vi "Initialize Attributes.vi"(8 "error in (no error)":errorcluster, 10 "Attribute Data":variant, 11 "BNT_DSCXYGraph in":refnum<class "BNT_DSCXYGraph.lvclass">) -> (0 "error out":errorcluster, 2 "Found?":bool, 3 "BNT_DSCXYGraph out":refnum<class "BNT_DSCXYGraph.lvclass">)   [LabVIEW 2015, in "BNT_DSCXYGraph.lvlib" / "BNT_DSCXYGraph.lvclass"]
doc: "Initialize object attribute.\n\nUnique resources should be allocated elsewhere!"
uses:
  BNT_DSCXYGraph.lvclass
  BNT_DSCXYGraph.lvclass/BNT_DSCXYGraph.ctl
  CSPP_Core/Actors/CS++GUIActor/CS++GUIActor.lvclass
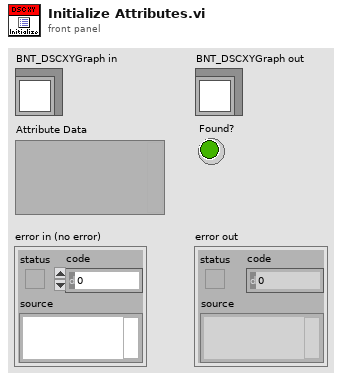
[diagram p1: front panel]
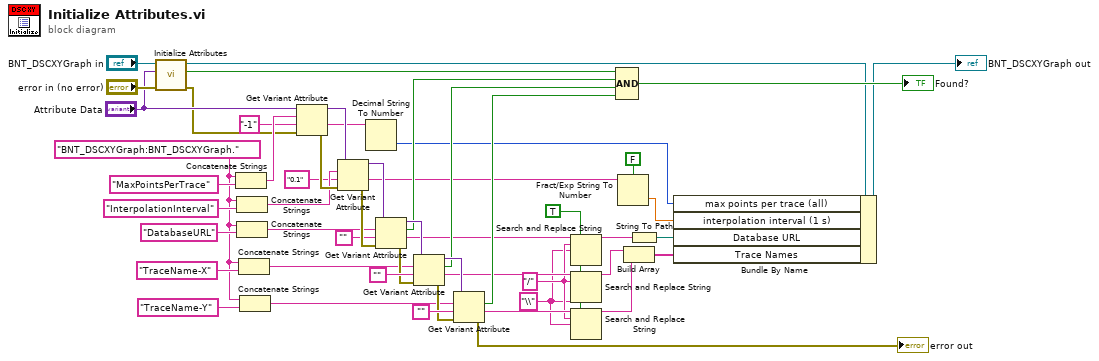
[diagram p0: block diagram]
diagram:
  w3 = TRUE ("replace all? (F)")
  w1 = "\\" ("replace string (\"\")")
  w2 = "/" ("search string")
  w38 = "BNT_DSCXYGraph:BNT_DSCXYGraph."
  n1 = call-parent "Initialize Attributes.vi"("error in (no error)"="error in (no error)", "Attribute Data"="Attribute Data", "CS++GUIActor in"="BNT_DSCXYGraph in") -> ("error out"=w44:errorcluster, "Found?"=w45:bool, "CS++GUIActor out"=w11:refnum<class "BNT_DSCXYGraph.lvclass">)  [unwired: 6 in]
  n2 = Concatenate Strings(w38, "MaxPointsPerTrace" ("string")) -> (w50:string)
  n3 = Concatenate Strings(w38, "InterpolationInterval" ("string")) -> (w47:string)
  n4 = Concatenate Strings(w38, "DatabaseURL" ("string")) -> (w33:string)
  n5 = Concatenate Strings(w38, "TraceName-X" ("string")) -> (w28:string)
  n6 = Concatenate Strings(w38, "TraceName-Y" ("string")) -> (w24:string)
  n7 = Get Variant Attribute(Variant="Attribute Data", name=w50, default value (empty Variant)="-1" ("string"), error in=w44) -> (duplicate Variant=w49:variant, value=w16:string, error out=w48:errorcluster)  [unwired: 1 out]
  n8 = Get Variant Attribute(Variant=w49, name=w47, default value (empty Variant)="0.1" ("string"), error in=w48) -> (duplicate Variant=w35:variant, value=w14:string, error out=w34:errorcluster)  [unwired: 1 out]
  n9 = Decimal String To Number(string=w16) -> (number=w15:i32)  [unwired: 2 in, 1 out]
  n10 = Get Variant Attribute(Variant=w35, name=w33, default value (empty Variant)="", error in=w34) -> (duplicate Variant=w30:variant, found=w23:bool, value=w4:string, error out=w29:errorcluster)
  n11 = Get Variant Attribute(Variant=w30, name=w28, default value (empty Variant)="", error in=w29) -> (duplicate Variant=w25:variant, found=w22:bool, value=w9:string, error out=w26:errorcluster)
  n12 = Get Variant Attribute(Variant=w25, name=w24, default value (empty Variant)="", error in=w26) -> (found=w21:bool, value=w7:string, error out=→"error out":errorcluster)  [unwired: 1 out]
  n13 = Search and Replace String(replace all?=w3, input string=w4, search string=w2, replace string=w1) -> (result string=w5:string)  [unwired: 4 in, 3 out]
  n14 = Search and Replace String(replace all?=w3, input string=w9, search string=w2, replace string=w1) -> (result string=w8:string)  [unwired: 4 in, 3 out]
  n15 = Search and Replace String(replace all?=w3, input string=w7, search string=w2, replace string=w1) -> (result string=w6:string)  [unwired: 4 in, 3 out]
  n16 = Compound Arithmetic op=AND(w45, w23, w22, w21) -> (→"Found?":bool)
  n17 = Fract/Exp String To Number(use system decimal point (T)=FALSE, string=w14) -> (number=w13:dbl)  [unwired: 2 in, 1 out]
  n18 = Build Array(w8, w6) -> (w17:string[])
  n19 = String To Path(string=w5) -> (path=w18:path)
  n20 = Bundle By Name(cluster=w11, "max points per trace (all)"=w15, "interpolation interval (1 s)"=w13, "Database URL"=w18, "Trace Names"=w17) -> (→"BNT_DSCXYGraph out":refnum<class "BNT_DSCXYGraph.lvclass">)
